vi "get tilt state.vi"(8 "error in (no error)":errorcluster, 11 "index":i32) -> (0 "error out":errorcluster, 3 "Output":T1)   [LabVIEW 2017, in "libfreenect.lvlib"]
doc: "EXPORT freenect_raw_tilt_state *freenect_lv_get_tilt_state(int index);"
uses:
  libfreenect.lvlib
  <vilib>/Utility/importsl/GetValueByPointer/GetValueByPointer.xnode
  <resource>/lvimptsl.dll
  freenect_lv.dll
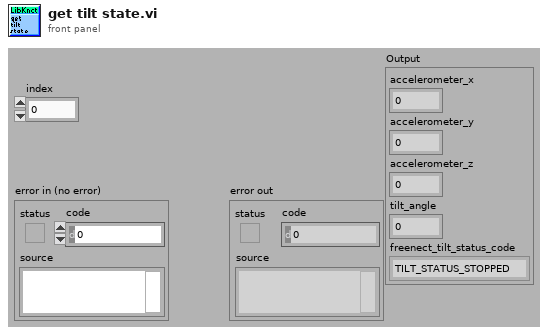
[diagram p1: front panel]
types:
  T1 = cluster{"accelerometer_x":i16, "accelerometer_y":i16, "accelerometer_z":i16, "tilt_angle":i8, "freenect_tilt_status_code":enum8{"TILT_STATUS_STOPPED", "TILT_STATUS_LIMIT", "UNUSED 1", "UNUSED 2", "TILT_STATUS_MOVING"}}
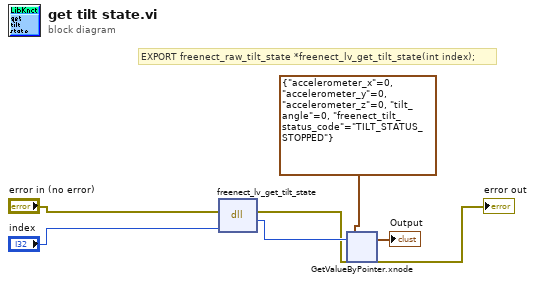
[diagram p0: block diagram]
diagram:
  # "EXPORT freenect_raw_tilt_state *freenect_lv_get_tilt_state(int index);"
  n1 = dll-call lib="C:/Users/Mats/Desktop/Bacheler prosjekt/Labview/Occupancy Grid Map Code - With model/freenect_lv.*" fn="freenect_lv_get_tilt_state"(error in="error in (no error)", "index"="index") -> (error out=w2:errorcluster, "return type"=w5:i32)  [unwired: 3 in, 1 out]
  n2 = xnode "GetValueByPointer.xnode"("Pointer"=w5, "InputType"=T1 {"accelerometer_x"=0, "accelerometer_y"=0, "accelerometer_z"=0, "tilt_angle"=0, "freenect_tilt_status_code"=enum."TILT_STATUS_STOPPED"} ("freenect_raw_tilt_state"), "ErrorIn"=w2) -> ("Output"=→"Output":T1, "ErrorOut"=→"error out":errorcluster)  [unwired: 1 in]
